vi "清除产品ID.vi"(8 "error in (no error)":errorcluster, 11 "芯片编码":string) -> (0 "error out":errorcluster)   [LabVIEW 2013]
uses:
  <vilib>/Utility/error.llb/whitespace.ctl
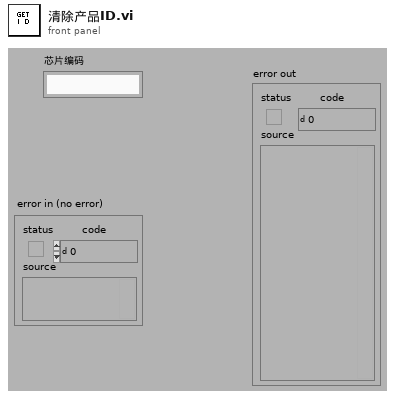
[diagram p1: front panel]
types:
  T1 = typedef "whitespace.ctl" = u16
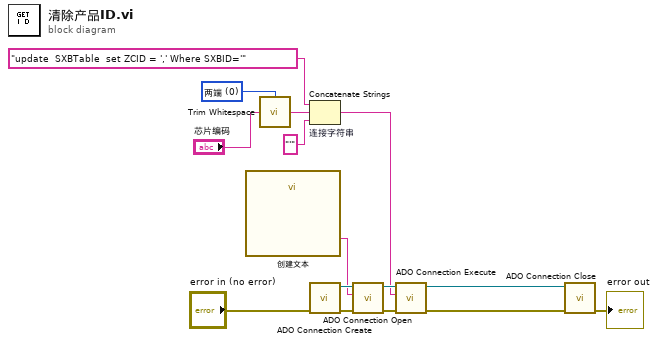
[diagram p0: block diagram]
diagram:
  w7 = T1 0 items=["两端", "字符串首端", "字符串末端"] ("location (both)")
  n1 = call "创建文本"() -> ("Result"=w1:string)  [unwired: 14 in, 1 out]
  n2 = call <vilib>:"Trim Whitespace.vi"("string"="芯片编码", "location (both)"=w7) -> ("trimmed string"=w8:string)
  n3 = Concatenate Strings "连接字符串"("update  SXBTable  set ZCID = ',' Where SXBID='" ("字符串 2"), w8, "'" ("字符串 2")) -> (w6:string)
  n4 = call "ADO Connection Create.vi"("error in (no error)"="error in (no error)") -> ("error out"=w14:errorcluster, "ADODB._Connection Out"=w15:refnum<k7>)  [unwired: 9 out]
  n5 = call "ADO Connection Open.vi"("error in (no error)"=w14, "ConnectionString"=w1, "ADODB._Connection In"=w15) -> ("error out"=w13:errorcluster, "ADODB._Connection Out"=w12:refnum<k7>)  [unwired: 7 out]
  n6 = call "ADO Connection Execute.vi"("error in (no error)"=w13, "CommandText"=w6, "ADODB._Connection In"=w12) -> ("error out"=w2:errorcluster, "ADODB._Connection Out"=w11:refnum<k7>)  [unwired: 7 out]
  n7 = call "ADO Connection Close.vi"("error in (no error)"=w2, "ADODB._Connection In"=w11) -> ("error out"=→"error out":errorcluster)  [unwired: 9 out]
